vi "OAT Remove Baseline.vi"(8 "error in (no error)":errorcluster, 10 "baseline in":cluster{"r0":dbl, "dr":dbl, "Y":dbl[]}={"r0"=0.0, "dr"=1.0, "Y"=[]} {"r0" format="%.2p"; "dr" format="%.2p"; "Y" format="%.2f"}, 11 "resampled signal in":cluster{"r0":dbl, "dr":dbl, "Y":dbl[]}={"r0"=0.0, "dr"=1.0, "Y"=[]} {"r0" format="%.2p"; "dr" format="%.2p"; "Y" format="%.2f"}) -> (0 "error out":errorcluster, 3 "compensated signal":cluster{"r0":dbl, "dr":dbl, "Y":dbl[]}={"r0"=0.0, "dr"=1.0, "Y"=[]} {"r0" format="%.2p"; "dr" format="%.2p"; "Y" format="%.2f"})   [LabVIEW 2017]
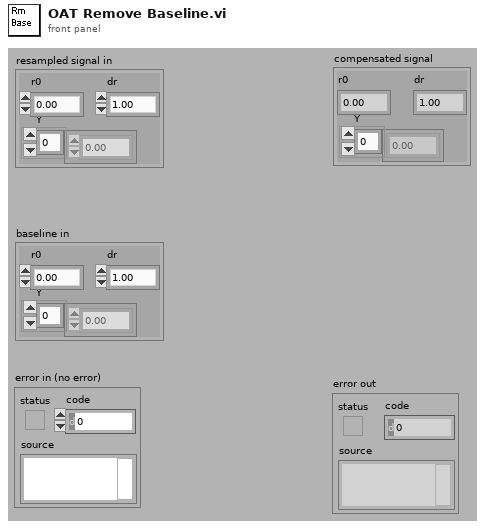
[diagram p1: front panel]
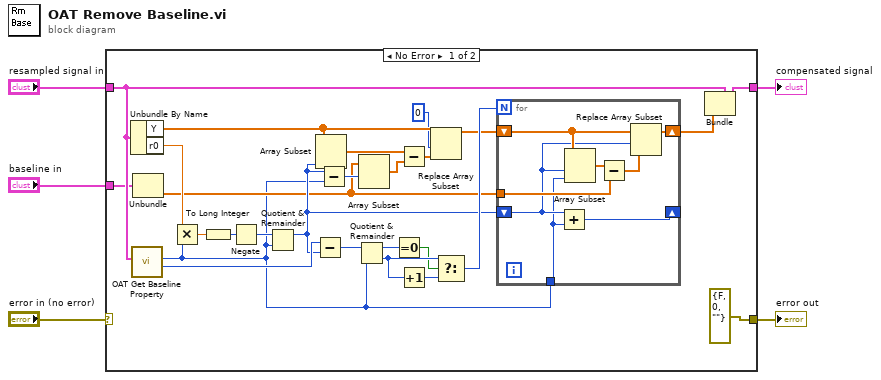
[diagram p0: block diagram]
diagram:
  n1 = case shown="No Error" "error in (no error)" {
    selector: "error in (no error)" -> [_ w40]
    tunnel: [w31 w41] -> w1
    tunnel: "resampled signal in" -> [w23 w41]
    tunnel: [errorcluster {"status"=FALSE, "code"=0, "source"=""} ("error IO") w40] -> w3
    tunnel: "baseline in" -> [w22 _]
    frame No Error {
      n2 = Unbundle By Name(w23) -> ("Y"=w18:dbl[], "r0"=w21:dbl)
      n3 = call <vilib>:"OAT Get Baseline Property.vi"("baseline"=w23) -> ("samples"=w15:i32, "samples/rev"=w6:i32)  [unwired: 9 in]
      n4 = Unbundle(w22) -> ("Y"=w8:dbl[])  [unwired: 2 out]
      n5 = Multiply(x=w21, y=w6) -> (x*y=w20:dbl)
      n6 = To Long Integer(number=w20) -> (32bit integer=w19:i32)
      n7 = Negate(x=w19) -> (-x=w13:i32)
      n8 = Quotient & Remainder(x=w13, y=w6) -> (x-y*floor(x/y)=w10:i32)  [unwired: 1 out]
      n9 = Subtract(x=w15, y=w10) -> (x-y=w14:i32)
      n10 = Array Subset(array=w18, length=w10) -> (w12:dbl[])  [unwired: 1 in]
      n11 = Subtract(x=w10, y=w6) -> (x-y=w9:i32)
      n12 = Quotient & Remainder(x=w14, y=w6) -> (x-y*floor(x/y)=w28:i32, floor(x/y)=w30:i32)
      n13 = Array Subset(array=w8, index=w9) -> (w11:dbl[])  [unwired: 1 in]
      n14 = Equal To 0?(x=w28) -> (x = 0?=w27:bool)
      n15 = Subtract(x=w12, y=w11) -> (x-y=w7:dbl[])
      n16 = Increment(x=w30) -> (x+1=w29:i32)
      n17 = Replace Array Subset(array=w18, new element=w7, index=0) -> (w16:dbl[])
      n18 = Select(t=w30, s=w27, f=w29) -> (s? t:f=w26:i32)
      n19 = for {
        N: w26 -> [_]
        shift-right: [w36] -> w25
        shift-left: w16 -> [w37]
        tunnel: w6 -> [w33]
        tunnel: w8 -> [w35]
        shift-right: [w32] -> _
        shift-left: w10 -> [w34]
        n20 = Add(x=w34, y=w33) -> (x+y=w32:i32)
        n21 = Array Subset(array=w37, index=w34, length=w33) -> (w39:dbl[])
        n22 = Subtract(x=w39, y=w35) -> (x-y=w38:dbl[])
        n23 = Replace Array Subset(array=w37, new element=w38, index=w34) -> (w36:dbl[])
      }
      n24 = Bundle(cluster=w23, "Y"=w25) -> (w31:cluster{"r0":dbl, "dr":dbl, "Y":dbl[]})  [unwired: 2 in]
    }
    frame Error {
    }
  }
  "error out" <- w3
  "compensated signal" <- w1
